vi "GFITS_GetImList.vi"(8 "error in (no error)":errorcluster, 11 "Path":path=path "/home/ArcVIEW/Modules/Database/private/vis/imlist.log") -> (0 "error out":errorcluster, 2 "answer":string, 3 "list":string[][](array[string]))   [LabVIEW 2016]
uses:
  <vilib>/Utility/config.llb/Read Key (String).vi
  <vilib>/Utility/config.llb/NI_LVConfig.lvlib
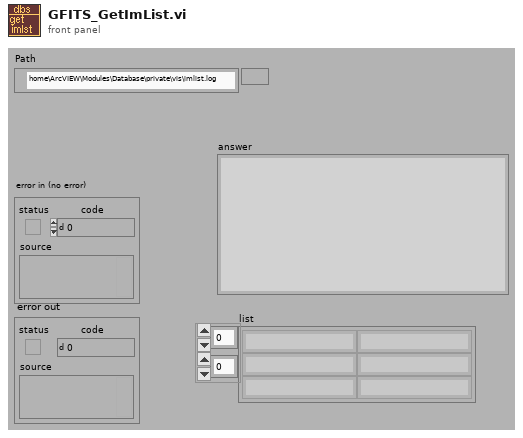
[diagram p1: front panel]
types:
  T1 = typedef "NI_LVConfig.lvlib/Config Data RefNum.ctl" = refnum<k1>
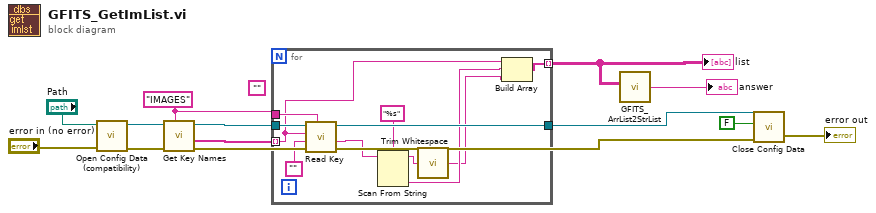
[diagram p0: block diagram]
diagram:
  (unwired) ""
  w8 = "IMAGES" ("section")
  n1 = call <vilib>:"Open Config Data (compatibility).vi"("error in (no error)"="error in (no error)", "configuration file path"="Path") -> ("error out"=w10:errorcluster, "refnum"=w9:T1)  [unwired: 7 in, 1 out]
  n2 = call <vilib>:"Get Key Names.vi"("section"=w8, "error in (no error)"=w10, "refnum"=w9) -> ("error out"=w6:errorcluster, "key names"=w4:string[], "refnum out"=w7:T1)  [unwired: 6 out]
  n3 = for {
    tunnel: w4 -> [w20] mode=indexing
    tunnel: w8 -> [w24]
    tunnel: w7 -> [w23]
    tunnel: [w21] -> w5
    tunnel: [w19] -> w3 mode=indexing
    n4 = call-poly <vilib>:"Read Key.vi"("section"=w24, "default value"="", "key"=w20, "refnum"=w23) -> ("value"=w16:string, "refnum out"=w21:T1)  [unwired: 2 in, 4 out]
    n5 = Scan From String(format string="%s", input string=w16) -> (remaining string=w18:string, output 1=w15:string)  [unwired: 2 in, 3 out]
    n6 = call <vilib>:"Trim Whitespace.vi"("string"=w18) -> ("trimmed string"=w14:string)  [unwired: 1 in]
    n7 = Build Array(w20, w15, w14) -> (w19:string[])
  }
  "list" <- w3
  n8 = call "GFITS_ArrList2StrList.vi"("List In"=w3) -> ("List Out"=→"answer":string)  [unwired: 9 out]
  n9 = call <vilib>:"Close Config Data.vi"("error in (no error)"=w6, "write file if changed (T)"=FALSE ("write configuration file? (T)"), "refnum"=w5) -> ("error out"=→"error out":errorcluster)  [unwired: 8 out]
